vi "GSI-HVSwitch2.constructor.vi"(0 "name":string, 2 "data in":string, 5 "error in (no error)":errorcluster) -> (14 "i ref out":refnum<vi>, 16 "data out":string, 19 "error out":errorcluster)   [LabVIEW 2014, in "GSI-HVSwitch2.lvlib"]
doc: "Constructor of the GSI-HVSwitch2 class.\n\nauthor: Dietrich Beck, GSI\nmaintainer: Dietrich Beck, GSI\nhistory: \n08-JUL-2005, created\n30-OCT-2006, migrated to CS 3.00\n\nLicense Agreement for this software:\n\nCopyright (C)\nGesellschaft für Schwerionenforschung, GSI\nPlanckstr. 1\n64291 Darmstadt\nGermany\n\nContact: D.Beck@gsi.de \n\nThis program is free software; you can redistribute it and/or modify it under the terms of the \nGNU General Public License as published by the Free Software Foundation; either version 2 of \nthe license, or (at your option) any later version.\n\nThis program is distributed in the hope that it will be useful, but WITHOUT ANY WARRANTY; \nwithout even the implied warranty of MERCHANTABILITY or FITNESS FOR A PARTICULAR PURPOSE. See the GNU General License for more details (http://www.gnu.org).\n\nGesellschaft für Schwerionenforschung, GSI\nPlanckstr. 1, 64291 Darmstadt, Germany\nFor all questions and ideas contact: M.Richter@gsi.de, H.Brand@gsi.de or D.Beck@gsi.de.\nLast update: 16-JUN-2004"
uses:
  GSI-HVSwitch2.lvlib
  CS_Core/CSApplicationBaseClasses/DeviceBase/DeviceBase.myEventNames.ctl
  CS_Core/CSApplicationBaseClasses/PSChannelBase/PSChannelBase.myEventNames.ctl
  GSI-HVSwitch2.mode.ctl
  CS_Core/BaseProcess/BaseProcess.lvlib
  CS_Core/CSSystem/CSSystemLib/CSSystemLib.lvlib
  CSlibraries-extern/DimLVEvent/LVDimInterface/LVDimInterface.lvlib
  CS_Core/CSApplicationBaseClasses/PSChannelBase/PSChannelBase.lvlib
  CS_Core/CSApplicationBaseClasses/DeviceBase/DeviceBase.lvlib
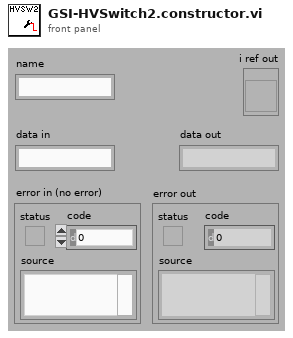
[diagram p1: front panel]
types:
  T1 = typedef "GSI-HVSwitch2.lvlib/GSI-HVSwitch2.mode.ctl" = enum16{"unknown", "switch", "stepper"}
  T2 = enum16{"SetAttribute", "GetAttribute", "CreateAttribute", "DestroyAttribute", "DestroyAllAtributes"}
  T3 = typedef "PSChannelBase.lvlib/PSChannelBase.myEventNames.ctl" = enum16{"lvmsg://EmergencyOff", "lvmsg://SetOnOff", "lvmsg://GetOnOff", "lvmsg://SetVoltage", "lvmsg://GetVoltage", "lvmsg://SetCurrent", "lvmsg://GetCurrent", "lvmsg://SetTripCurrent", "lvmsg://GetTripCurrent", "lvmsg://SetRampUpSpeed", "lvmsg://GetRampUpSpeed", "lvmsg://SetRampDownSpeed", "lvmsg://GetRampDownSpeed", "lvmsg://SetChannelOnOff", "lvmsg://GetChannelOnOff", "lvmsg://SetChannelVoltage", "lvmsg://GetChannelVoltage", "lvmsg://SetChannelCurrent", "lvmsg://GetChannelCurrent", "lvmsg://SetChannelTripCurrent", "lvmsg://GetChannelTripCurrent", "lvmsg://SetChannelRampUpSpeed", "lvmsg://GetChannelRampUpSpeed", "lvmsg://SetChannelRampDownSpeed", "lvmsg://GetChannelRampDownSpeed"}
  T4 = typedef "DeviceBase.lvlib/DeviceBase.myEventNames.ctl" = enum16{"lvmsg://Initialize", "lvmsg://Close", "lvmsg://Configure", "lvmsg://Reset", "lvmsg://IDQuery"}
  T5 = typedef "GSI-HVSwitch2.lvlib/GSI-HVSwitch2.i attribute.ctl" = cluster{"SDEX VISA Cluster":T6, "SetVoltage SW0":dbl, "SetVoltage SW1":dbl, "ActTempAmp":dbl, "ActTempPS1":dbl, "ActTempPS2":dbl, "mode":T1, "interfaceInitialized":bool, "serviceIDs":cluster{"nomVoltage0ID":i32, "nomVoltage1ID":i32, "actTempAmpID":i32, "actTempPS1ID":i32, "actTempPS2ID":i32, "modeID":i32}, "usedChannels":i32}
  T6 = typedef "SDEXDriver.lvlib/SDEX.VISA Control.ctl" = cluster{"VISA resource name":refnum<visa-resource-name>, "HEX address":u16, "VISA Timeout Value (1000 ms)":u32, "Lock Timeout (1000 ms)":u32, "semaphore":T7, "Baud rate":u32, "revision":T8, "deviceInfo":string}
  T7 = typedef "Semaphore RefNum" = refnum<k1>
  T8 = typedef "SDEXDriver.lvlib/SDEX.revisionType.ctl" = enum16{"unknown", "hvamp3", "hvswi1", "htrp0", "WDG0"}
  T9 = typedef "BaseProcess.lvlib/BaseProcess.i attribute.ctl" = cluster{"EventStatus":string, "EventError":i32, "PresetEvtWatchD":i32, "PresetPdcWatchD":i32, "EventTimeout":i32, "PeriodicInterval":i32, "Interface":string[], "Address":string[], "Special":string[], "PeriodicError":i32, "PeriodicStatus":string, "SuperProc":string, "Descriptors":T10[], "CaseRef":refnum<vi>, "PdcRef":refnum<vi>, "Thread Ref":refnum<vi>, "eventErrorID":i32, "eventStatusID":i32, "periodicErrorID":i32, "periodicStatusID":i32, "pdcCtrID":i32}
  T10 = typedef "BaseProcess.lvlib/BaseProcess.descriptor definition.ctl" = cluster{"selector":string, "descriptor":T11}
  T11 = typedef "BaseProcess.lvlib/BaseProcess.descriptor string definition.ctl" = string
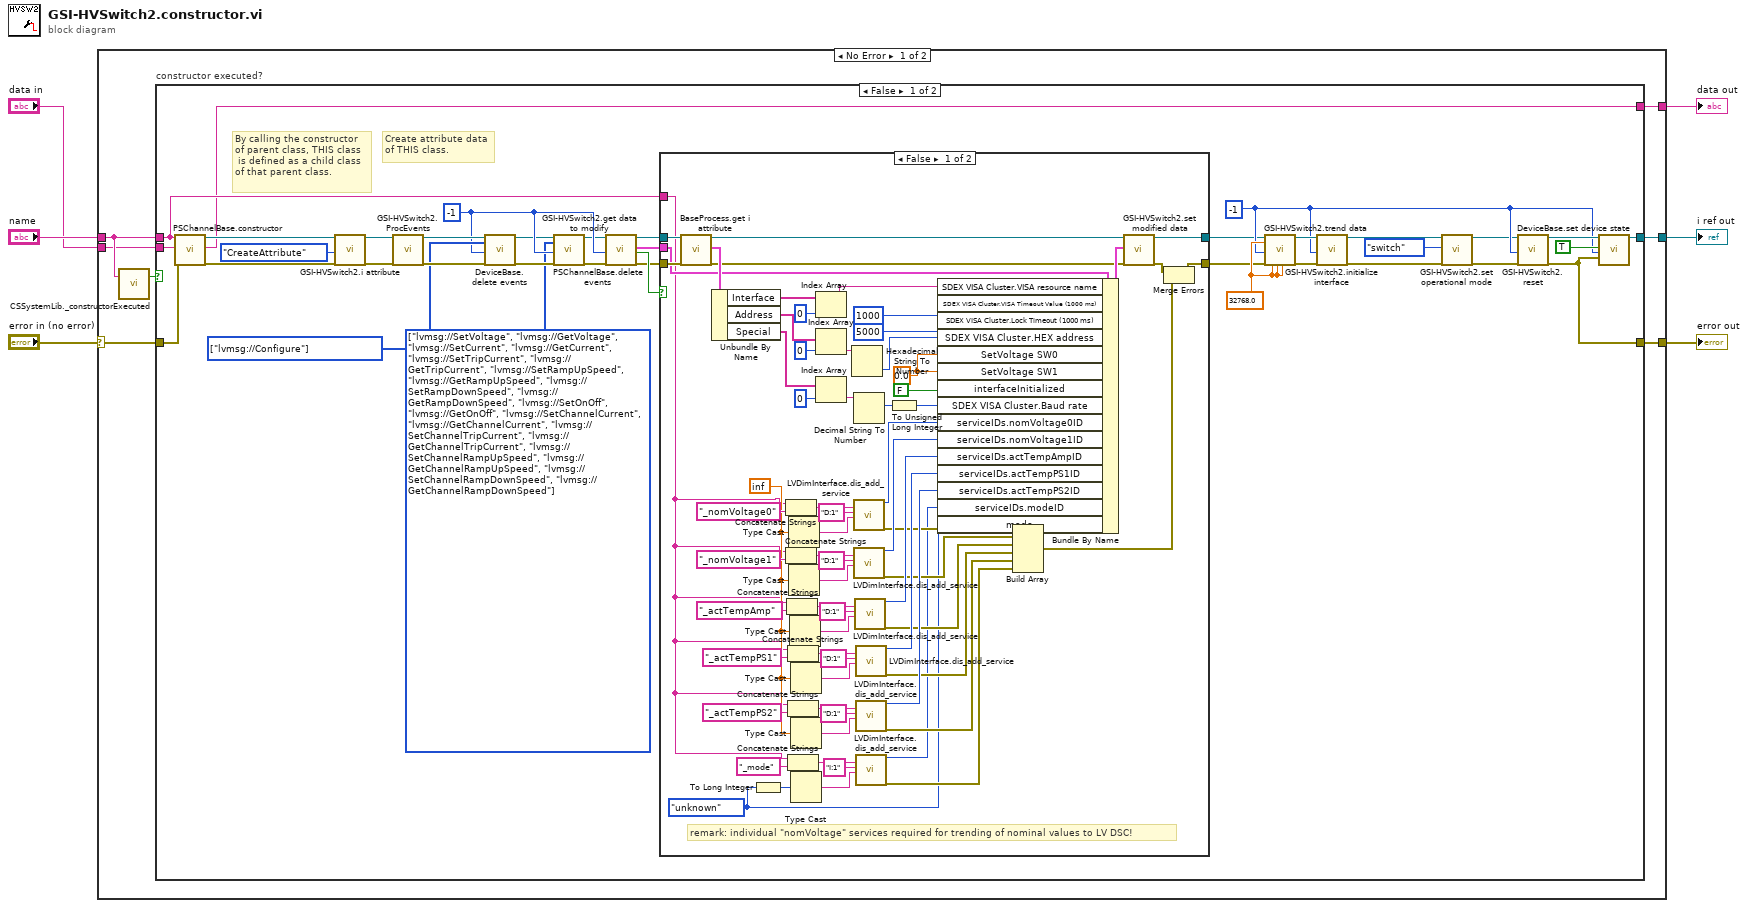
[diagram p0: block diagram]
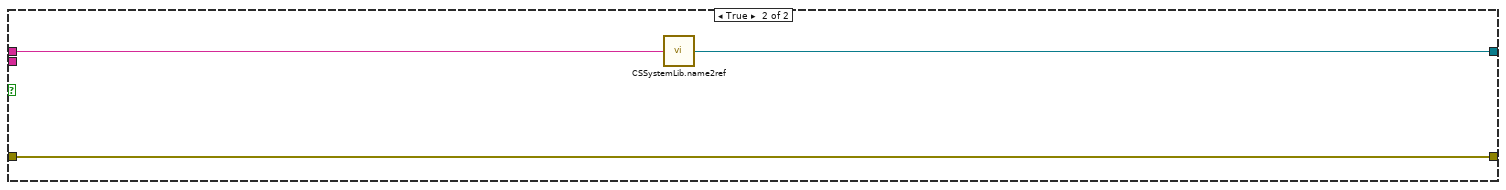
[diagram p3: hidden frame]
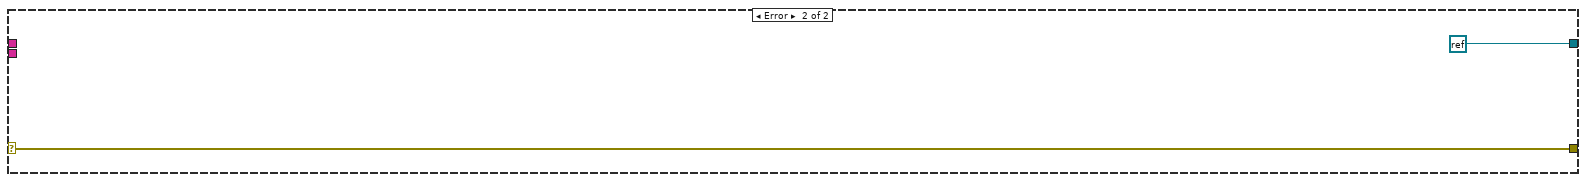
[diagram p4: hidden frame]
diagram:
  n1 = case shown="No Error" "error in (no error)" {
    selector: "error in (no error)" -> [w11 w123]
    tunnel: "name" -> [w9 _]
    tunnel: [w13 refnum<k0> refnum ("Not a Refnum Constant")] -> w5
    tunnel: [w12 w123] -> w4
    tunnel: "data in" -> [w8 _]
    tunnel: [w7 _] -> w1
    frame No Error {
      n2 = call "CSSystemLib._constructorExecuted.vi"("name"=w9) -> ("constructor executed?"=w10:bool)  [unwired: 18 in]
      n3 = case "constructor executed?" shown="False" w10 {
        tunnel: [w39 w121] -> w13
        tunnel: [w25 w120] -> w12
        tunnel: w11 -> [w40 w120]
        tunnel: w9 -> [w28 w122]
        tunnel: w8 -> [w23 _]
        tunnel: [w22 _] -> w7
        frame False {
          w29 = T3[] [enum."lvmsg://SetVoltage", enum."lvmsg://GetVoltage", enum."lvmsg://SetCurrent", enum."lvmsg://GetCurrent", enum."lvmsg://SetTripCurrent", enum."lvmsg://GetTripCurrent", enum."lvmsg://SetRampUpSpeed", enum."lvmsg://GetRampUpSpeed", enum."lvmsg://SetRampDownSpeed", enum."lvmsg://GetRampDownSpeed", enum."lvmsg://SetOnOff", enum."lvmsg://GetOnOff", enum."lvmsg://SetChannelCurrent", enum."lvmsg://GetChannelCurrent", enum."lvmsg://SetChannelTripCurrent", enum."lvmsg://GetChannelTripCurrent", enum."lvmsg://SetChannelRampUpSpeed", enum."lvmsg://GetChannelRampUpSpeed", enum."lvmsg://SetChannelRampDownSpeed", enum."lvmsg://GetChannelRampDownSpeed"] items=["lvmsg://EmergencyOff", "lvmsg://SetOnOff", "lvmsg://GetOnOff", "lvmsg://SetVoltage", "lvmsg://GetVoltage", "lvmsg://SetCurrent", "lvmsg://GetCurrent", "lvmsg://SetTripCurrent", "lvmsg://GetTripCurrent", "lvmsg://SetRampUpSpeed", "lvmsg://GetRampUpSpeed", "lvmsg://SetRampDownSpeed", "lvmsg://GetRampDownSpeed", "lvmsg://SetChannelOnOff", "lvmsg://GetChannelOnOff", "lvmsg://SetChannelVoltage", "lvmsg://GetChannelVoltage", "lvmsg://SetChannelCurrent", "lvmsg://GetChannelCurrent", "lvmsg://SetChannelTripCurrent", "lvmsg://GetChannelTripCurrent", "lvmsg://SetChannelRampUpSpeed", "lvmsg://GetChannelRampUpSpeed", "lvmsg://SetChannelRampDownSpeed", "lvmsg://GetChannelRampDownSpeed"] ("events")
          w35 = T4[] [enum."lvmsg://Configure"] items=["lvmsg://Initialize", "lvmsg://Close", "lvmsg://Configure", "lvmsg://Reset", "lvmsg://IDQuery"] ("events")
          w21 = -1
          w41 = 32768.0
          w33 = -1 ("ms timeout (10000)")
          # "Create attribute data\nof THIS class."
          # "By calling the constructor\nof parent class, THIS class\n is defined as a child class\nof that parent class."
          n4 = call "PSChannelBase.constructor.vi"("name"=w28, "data in"=w23, "error in (no error)"=w40) -> ("i ref out"=w50:refnum<vi>, "data out"=w22:string, "error out"=w49:errorcluster)  [unwired: 14 in]
          n5 = call "GSI-HVSwitch2.i attribute.vi"("VI Refnum"=w50, "Action"=T2."CreateAttribute", "error in (no error)"=w49) -> ("VI Refnum out"=w47:refnum<vi>, "error out"=w46:errorcluster)  [unwired: 14 in, 1 out]
          n6 = call "GSI-HVSwitch2.ProcEvents.vi"("i ref in"=w47, "error in (no error)"=w46) -> ("i ref out"=w36:refnum<vi>, "error out"=w37:errorcluster)  [unwired: 16 in]
          n7 = call "DeviceBase.delete events.vi"("i ref in"=w36, "events"=w35, "ms timeout (10000)"=w33, "error in (no error)"=w37) -> ("i ref out"=w32:refnum<vi>, "error out"=w34:errorcluster)  [unwired: 13 in, 1 out]
          n8 = call "PSChannelBase.delete events.vi"("i ref in"=w32, "events"=w29, "ms timeout (10000)"=w33, "error in (no error)"=w34) -> ("i ref out"=w31:refnum<vi>, "error out"=w30:errorcluster)  [unwired: 13 in, 1 out]
          n9 = call "GSI-HVSwitch2.get data to modify.vi"("i ref in"=w31, "ms timeout (10000)"=w33, "error in (no error)"=w30) -> ("i ref out"=w43:refnum<vi>, "i attribute"=w42:T5, "timed out"=w45:bool, "error out"=w44:errorcluster)  [unwired: 13 in]
          n10 = case shown="False" w45 {
            tunnel: [w63 w119] -> w19
            tunnel: w44 -> [w116 w119]
            tunnel: [w103 w118] -> w18
            tunnel: w43 -> [w117 w118]
            tunnel: w42 -> [w110 _]
            tunnel: w28 -> [w52 _]
            frame False {
              w51 = GSI-HVSwitch2.mode."unknown" ("mode")
              w60 = 0.0 ("SetVoltage SW1")
              w62 = inf ("Positive Infinity")
              # "remark: individual \"nomVoltage\" services required for trending of nominal values to LV DSC!"
              n11 = call "BaseProcess.get i attribute.vi"("i ref in"=w117, "error in (no error)"=w116) -> ("i ref out"=w104:refnum<vi>, "i attribute"=w115:T9, "error out"=w105:errorcluster)  [unwired: 15 in]
              n12 = Unbundle By Name(w115) -> ("Interface"=w114:string[], "Address"=w113:string[], "Special"=w99:string[])
              n13 = To Long Integer(number=w51) -> (32bit integer=w55:i32)
              n14 = Concatenate Strings(w52, "_nomVoltage0" ("string")) -> (w94:string)
              n15 = Concatenate Strings(w52, "_nomVoltage1" ("string")) -> (w87:string)
              n16 = Concatenate Strings(w52, "_actTempAmp" ("string")) -> (w82:string)
              n17 = Concatenate Strings(w52, "_actTempPS1" ("string")) -> (w80:string)
              n18 = Concatenate Strings(w52, "_actTempPS2" ("string")) -> (w72:string)
              n19 = Concatenate Strings(w52, "_mode" ("string")) -> (w59:string)
              n20 = Type Cast(x=w62) -> (*(type *) &x=w91:string)  [unwired: 1 in]
              n21 = Type Cast(x=w62) -> (*(type *) &x=w90:string)  [unwired: 1 in]
              n22 = Type Cast(x=w62) -> (*(type *) &x=w85:string)  [unwired: 1 in]
              n23 = Type Cast(x=w62) -> (*(type *) &x=w77:string)  [unwired: 1 in]
              n24 = Type Cast(x=w62) -> (*(type *) &x=w75:string)  [unwired: 1 in]
              n25 = Type Cast(x=w55) -> (*(type *) &x=w56:string)  [unwired: 1 in]
              n26 = Index Array(array=w114, index=0) -> (element=w61:string)
              n27 = Index Array(array=w113, index=0) -> (element=w109:string)
              n28 = Index Array(array=w99, index=0) -> (element=w98:string)
              n29 = Hexadecimal String To Number(string=w109) -> (number=w100:u32)  [unwired: 2 in, 1 out]
              n30 = Decimal String To Number(string=w98) -> (number=w97:i32)  [unwired: 2 in, 1 out]
              n31 = call "LVDimInterface.dis_add_service.vi"("serviceName"=w94, "typeDescriptor"="D:1", "data"=w91) -> ("my_serviceID"=w95:i32, "error out"=w70:errorcluster)  [unwired: 15 in]
              n32 = call "LVDimInterface.dis_add_service.vi"("serviceName"=w87, "typeDescriptor"="D:1", "data"=w90) -> ("my_serviceID"=w86:i32, "error out"=w69:errorcluster)  [unwired: 15 in]
              n33 = call "LVDimInterface.dis_add_service.vi"("serviceName"=w82, "typeDescriptor"="D:1", "data"=w85) -> ("my_serviceID"=w81:i32, "error out"=w68:errorcluster)  [unwired: 15 in]
              n34 = call "LVDimInterface.dis_add_service.vi"("serviceName"=w80, "typeDescriptor"="D:1", "data"=w77) -> ("my_serviceID"=w76:i32, "error out"=w67:errorcluster)  [unwired: 15 in]
              n35 = call "LVDimInterface.dis_add_service.vi"("serviceName"=w72, "typeDescriptor"="D:1", "data"=w75) -> ("my_serviceID"=w71:i32, "error out"=w66:errorcluster)  [unwired: 15 in]
              n36 = call "LVDimInterface.dis_add_service.vi"("serviceName"=w59, "typeDescriptor"="I:1", "data"=w56) -> ("my_serviceID"=w54:i32, "error out"=w53:errorcluster)  [unwired: 15 in]
              n37 = To Unsigned Long Integer(number=w97) -> (unsigned 32bit integer=w96:u32)
              n38 = Bundle By Name(cluster=w110, "SDEX VISA Cluster.VISA resource name"=w61, "SDEX VISA Cluster.VISA Timeout Value (1000 ms)"=u32 1000, "SDEX VISA Cluster.Lock Timeout (1000 ms)"=u32 5000, "SDEX VISA Cluster.HEX address"=w100, "SetVoltage SW0"=w60, "SetVoltage SW1"=w60, "interfaceInitialized"=FALSE ("interfaceOpened"), "SDEX VISA Cluster.Baud rate"=w96, "serviceIDs.nomVoltage0ID"=w95, "serviceIDs.nomVoltage1ID"=w86, "serviceIDs.actTempAmpID"=w81, "serviceIDs.actTempPS1ID"=w76, "serviceIDs.actTempPS2ID"=w71, "serviceIDs.modeID"=w54, "mode"=w51) -> (w106:T5)
              n39 = Build Array(w70, w69, w68, w67, w66, w53) -> (w64:errorcluster[])
              n40 = call "GSI-HVSwitch2.set modified data.vi"("i ref in"=w104, "i attribute"=w106, "error in (no error)"=w105) -> ("i ref out"=w103:refnum<vi>, "error out"=w65:errorcluster)  [unwired: 15 in]
              n41 = Merge Errors(w65, w64) -> (w63:errorcluster)
            }
            frame True {
            }
          }
          n42 = call "GSI-HVSwitch2.trend data.vi"("i ref in"=w18, "ActVoltage"=w41, "ms timeout (10000)"=w21, "error in (no error)"=w19, "ActTempAmp"=w41, "ActTempPS1"=w41, "ActTempPS2"=w41) -> ("i ref out"=w27:refnum<vi>, "error out"=w26:errorcluster)  [unwired: 10 in, 1 out]
          n43 = call "GSI-HVSwitch2.initialize interface.vi"("i ref in"=w27, "ms timeout (10000)"=w21, "error in (no error)"=w26) -> ("i ref out"=w16:refnum<vi>, "error out"=w17:errorcluster)  [unwired: 14 in, 1 out]
          n44 = call "GSI-HVSwitch2.set operational mode.vi"("i ref in"=w16, "mode"=GSI-HVSwitch2.mode."switch", "error in (no error)"=w17) -> ("i ref out"=w14:refnum<vi>, "error out"=w15:errorcluster)  [unwired: 14 in, 1 out]
          n45 = call "GSI-HVSwitch2.reset.vi"("i ref in"=w14, "ms timeout (10000)"=w21, "error in (no error)"=w15) -> ("i ref out"=w24:refnum<vi>, "error out"=w25:errorcluster)  [unwired: 14 in, 1 out]
          n46 = call "DeviceBase.set device state.vi"("i ref in"=w24, "implicit"=TRUE, "ms timeout (10000)"=w21, "device error"=w25) -> ("i ref out"=w39:refnum<vi>)  [unwired: 13 in, 2 out]
        }
        frame True {
          n47 = call "CSSystemLib.name2ref.vi"("name"=w122) -> ("obj refnum"=w121:refnum<vi>)
        }
      }
    }
    frame Error {
    }
  }
  "i ref out" <- w5
  "error out" <- w4
  "data out" <- w1
